vi "ShowDiff.vi"(0 "RawDiff":string, 1 "Alt.Name Old":string, 5 "Alt.Name New":string) -> (6 "UserDone":bool)   [LabVIEW 2013]
uses:
  <vilib>/Utility/miscctls.llb/LVRowAndColumnTypeDef.ctl
  <vilib>/Utility/miscctls.llb/LVRowAndColumnUnsignedTypeDef.ctl
panel:
  in  "Next Button":bool
  in  "Previous Button":bool
  in  "Done":bool
  out "Legend":string[][](table)
  out "FormattedDiff":string[][](table)
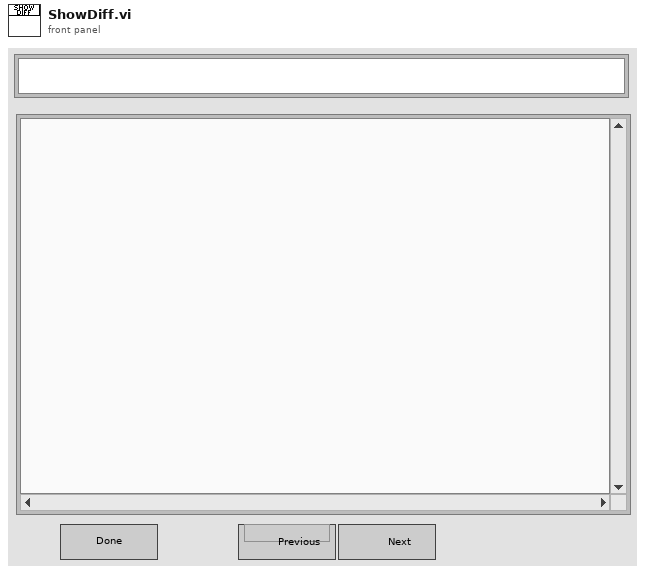
[diagram p1: front panel]
types:
  T1 = typedef "LVRowAndColumnTypeDef.ctl" = cluster{"Row":i32, "Column":i32}
  T2 = cluster{"left":i16, "top":i16, "right":i16, "bottom":i16}
  T3 = typedef "LVRowAndColumnUnsignedTypeDef.ctl" = cluster{"Row":u32, "Column":u32}
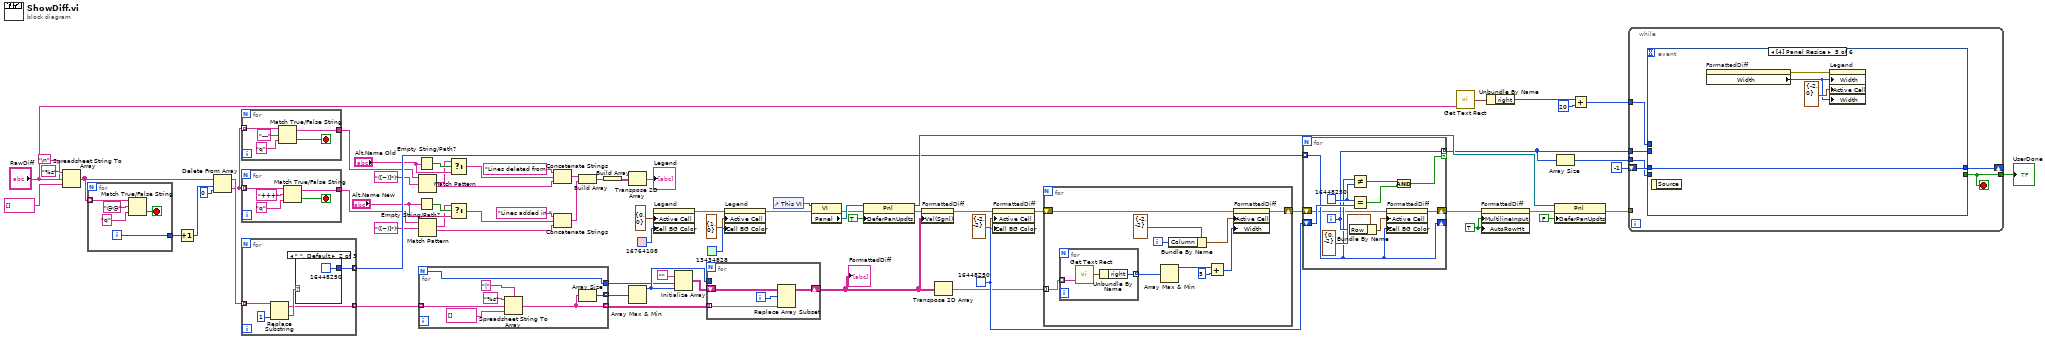
[diagram p0: block diagram]
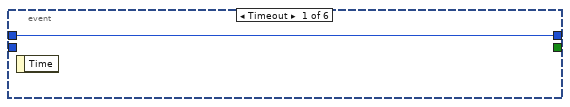
[diagram p2: hidden frame]
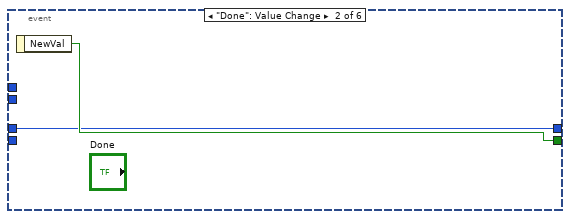
[diagram p3: hidden frame]
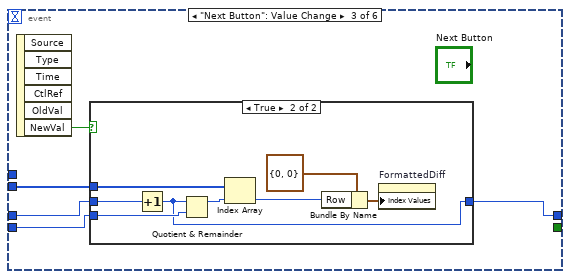
[diagram p4: hidden frame]
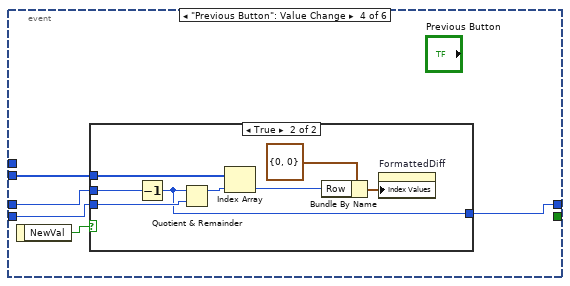
[diagram p6: hidden frame]
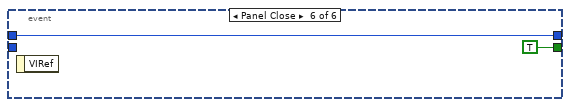
[diagram p8: hidden frame]
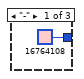
[diagram p9: hidden frame]
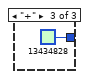
[diagram p10: hidden frame]
diagram:
  w59 = TRUE ("Multiple Line Input")
  w21 = u32 16448250
  n1 = Spreadsheet String To Array(delimiter (Tab)="\n", format string="%s", spreadsheet string="RawDiff", array type (2D Dbl)=string[] []) -> (array=w27:string[])
  n2 = for {
    tunnel: [w76] -> w26
    tunnel: w27 -> [w73] mode=indexing
    i -> [w76]
    stop <- w75 stop-if-true
    n3 = Match True/False String(2:"q" ("false string"), 3:"@@" ("true string"), 4:w73) -> (0:w75:bool)  [unwired: 1 out]
  }
  n4 = Increment(x=w26) -> (x+1=w25:i32)
  n5 = Delete From Array(array=w27, length=w25, index=0) -> (deleted portion=w23:string[], array with subset deleted=w62:string[])
  n6 = for {
    tunnel: w23 -> [w79] mode=indexing
    tunnel: [w77] -> w22
    stop <- w81 stop-if-true
    n7 = Match True/False String(2:"q" ("false string"), 3:"---" ("true string"), 4:w79) -> (0:w81:bool, 1:w77:string)
  }
  n8 = for {
    tunnel: w23 -> [w84] mode=indexing
    tunnel: [w82] -> w24
    stop <- w86 stop-if-true
    n9 = Match True/False String(2:"q" ("false string"), 3:"+++" ("true string"), 4:w84) -> (0:w86:bool, 1:w82:string)
  }
  n10 = for {
    tunnel: w62 -> [w91] mode=indexing
    tunnel: [w89] -> w58 mode=indexing
    tunnel: [w87] -> w13 mode=indexing
    n11 = Replace Substring(2:1 ("length (len. of substring)"), 5:w91) -> (0:w88:string, 1:w87:string)  [unwired: 2 in]
    n12 = case shown="\" \", Default" w88 {
      tunnel: [u32 16764108 u32 16448250 u32 13434828] -> w89
      frame "-" {
      }
      frame " ", Default {
      }
      frame "+" {
      }
    }
  }
  n13 = Empty String/Path?(string/path="Alt.Name Old") -> (empty?=w45:bool)
  n14 = Empty String/Path?(string/path="Alt.Name New") -> (empty?=w36:bool)
  n15 = Match Pattern(string=w22, regular expression="([~)]*)") -> (match substring=w43:string, after substring=w41:string)  [unwired: 1 in, 2 out]
  n16 = Match Pattern(string=w24, regular expression="([~)]*)") -> (match substring=w35:string, after substring=w31:string)  [unwired: 1 in, 2 out]
  n17 = for {
    N -> [w95]
    tunnel: w13 -> [w98] mode=indexing
    tunnel: [w99] -> w12 mode=indexing
    tunnel: [w96] -> w11 mode=indexing
    tunnel: [w95] -> w7
    n18 = Spreadsheet String To Array(delimiter (Tab)="|", format string="%s", spreadsheet string=w98, array type (2D Dbl)=string[] []) -> (array=w96:string[])
    n19 = Array Size(array=w96) -> (size(s)=w99:i32)
  }
  n20 = Select(t=w43, s=w45, f="Alt.Name Old") -> (s? t:f=w42:string)
  n21 = Select(t=w35, s=w36, f="Alt.Name New") -> (s? t:f=w32:string)
  n22 = Concatenate Strings("Lines deleted from " ("string"), w42, w41) -> (w39:string)
  n23 = Concatenate Strings("Lines added in " ("string"), w32, w31) -> (w34:string)
  n24 = Build Array(w39, w34) -> (w28:string[])
  n25 = Build Array(w28) -> (w29:string[][])
  n26 = Transpose 2D Array(2D array=w29) -> (transposed array=→"Legend":string[][])
  n27 = Array Max & Min(array=w12) -> (max value=w8:i32)  [unwired: 3 out]
  n28 = property on="Legend" class="Tbl (strict)"("Active Cell"=T1 {"Row"=0, "Column"=0} ("Active Cell:Active Cell"), "Cell BG Color"=u32 16764108) -> (error out=w47:errorcluster)  [unwired: 2 in, 1 out]
  n29 = Initialize Array("", w7, w8) -> (w9:string[][])
  n30 = for {
    tunnel: w8 -> [_]
    tunnel: w11 -> [w104] mode=indexing
    shift-right: [w102] -> w6
    shift-left: w9 -> [w105]
    i -> [w103]
    n31 = Replace Array Subset(array=w105, new element=w104, index (row)=w103) -> (w102:string[][])  [unwired: 1 in]
  }
  "FormattedDiff" <- w6
  n32 = property on="Legend" class="Tbl (strict)"(error in=w47, "Active Cell"=T1 {"Row"=1, "Column"=0} ("Active Cell:Active Cell"), "Cell BG Color"=u32 13434828) -> (error out=w17:errorcluster)  [unwired: 1 in, 1 out]
  n33 = control-ref of="This VI"() -> (w71:refnum<vi>)
  n34 = property class="VI"(reference=w71, error in=w17) -> (error out=w69:errorcluster, "Panel"=w70:refnum<vi>)  [unwired: 1 out]
  n35 = property on="Property Node" class="Pnl"(reference=w70, error in=w69, "DeferPanUpdts"=TRUE ("Defer Panel Updates")) -> (reference out=w67:refnum<vi>, error out=w14:errorcluster)
  n36 = property on="FormattedDiff" class="Tbl (strict)"(error in=w14, "Val(Sgnl)"=w6) -> (error out=w15:errorcluster)  [unwired: 1 in, 1 out]
  n37 = Transpose 2D Array(2D array=w6) -> (transposed array=w5:string[][])
  n38 = property on="FormattedDiff" class="Tbl (strict)"(error in=w15, "Active Cell"=T1 {"Row"=-2, "Column"=-2} ("Active Cell:Active Cell"), "Cell BG Color"=w21) -> (error out=w3:errorcluster)  [unwired: 1 in, 1 out]
  n39 = for {
    tunnel: w5 -> [w115] mode=indexing
    shift-right: [w106] -> w1
    shift-left: w3 -> [w107]
    i -> [w111]
    n40 = for {
      tunnel: w115 -> [w117] mode=indexing
      tunnel: [w116] -> w114 mode=indexing
      n41 = call <vilib>:"Get Text Rect.vi"("text"=w117) -> ("rect"=w118:T2)  [unwired: 8 in]
      n42 = Unbundle By Name(w118) -> ("right"=w116:i16)
    }
    n43 = Array Max & Min(array=w114) -> (max value=w110:i16)  [unwired: 3 out]
    n44 = Bundle By Name(cluster=T1 {"Row"=-2, "Column"=-2} ("Active Cell:Active Cell"), "Column"=w111) -> (w112:T1)
    n45 = Add(x=w110, y=i16 5) -> (x+y=w109:i16)
    n46 = property on="FormattedDiff" class="Tbl (strict)"(error in=w107, "Active Cell"=w112, "Width"=w109) -> (error out=w106:errorcluster)  [unwired: 1 in, 1 out]
  }
  n47 = for {
    shift-right: [w120] -> w2
    shift-left: w1 -> [w119]
    tunnel: w58 -> [w121] mode=indexing
    shift-right: [w121] -> _
    shift-left: w21 -> [w126]
    tunnel: [w123] -> w19 mode=indexing if=w122
    i -> [w123]
    w127 = u32 16448250
    n48 = Bundle By Name(cluster=T1 {"Row"=0, "Column"=-2} ("Active Cell:Active Cell"), "Row"=w123) -> (w128:T1)
    n49 = Not Equal?(x=w121, y=w127) -> (x != y?=w125:bool)
    n50 = Equal?(x=w127, y=w126) -> (x = y?=w124:bool)
    n51 = property on="FormattedDiff" class="Tbl (strict)"(error in=w119, "Active Cell"=w128, "Cell BG Color"=w121) -> (error out=w120:errorcluster)  [unwired: 1 in, 1 out]
    n52 = And(x=w125, y=w124) -> (x .and. y?=w122:bool)
  }
  n53 = call <vilib>:"Get Text Rect.vi"("text"="RawDiff") -> ("rect"=w54:T2)  [unwired: 8 in]
  n54 = property on="FormattedDiff" class="Tbl (strict)"(error in=w2, "MultilineInput"=w59, "AutoRowHt"=w59) -> (error out=w60:errorcluster)  [unwired: 1 in, 1 out]
  n55 = Unbundle By Name(w54) -> ("right"=w16:i16)
  n56 = property on="Property Node" class="Pnl"(reference=w67, error in=w60, "DeferPanUpdts"=FALSE ("Defer Panel Updates")) -> (error out=w57:errorcluster)  [unwired: 1 out]
  n57 = Array Size(array=w19) -> (size(s)=w18:i32)
  n58 = Add(x=w16, y=i16 20) -> (x+y=w52:i16)
  n59 = while {
    tunnel: w57 -> [_]
    tunnel: [w135] -> w56
    tunnel: w52 -> [w134]
    tunnel: w19 -> [w133]
    tunnel: w18 -> [w131]
    shift-right: [w130] -> _
    shift-left: -1 -> [w132]
    stop <- w135 stop-if-true
    n60 = event shown="[4] Panel Resize" {
      selector: _ -> [_ _ _ _ _ _]
      dyn-events: _ -> [_ _ _ _ _ _]
      timeout: _ -> [_ _ _ _ _ _]
      tunnel: [_ w138 _ _ _ TRUE ("NewVal")] -> w135
      tunnel: w134 -> [_ _ _ _ _ _]
      tunnel: w133 -> [_ _ w143 w157 _ _]
      tunnel: w132 -> [w136 w137 w141 w155 w168 w171]
      tunnel: w131 -> [_ _ w140 w154 _ _]
      tunnel: [w136 w137 w139 w153 w168 w171] -> w130
      event Timeout {
        n61 = event-data() -> ()  [unwired: 1 in, 1 out]
      }
      event "Done": Value Change {
        n62 = event-data() -> ("NewVal"=w138:bool)  [unwired: 1 in]
      }
      event "Next Button": Value Change {
        n63 = event-data() -> ("NewVal"=w142:bool)  [unwired: 1 in, 5 out]
        n64 = case shown="True" w142 {
          tunnel: w143 -> [_ w149]
          tunnel: w141 -> [w144 w148]
          tunnel: w140 -> [_ w147]
          tunnel: [w144 w145] -> w139
          frame False {
          }
          frame True {
            n65 = Increment(x=w148) -> (x+1=w145:i32)
            n66 = Quotient & Remainder(x=w145, y=w147) -> (x-y*floor(x/y)=w146:i32)  [unwired: 1 out]
            n67 = Index Array(array=w149, index=w146) -> (element=w150:i32)
            n68 = Bundle By Name(cluster=T3 {"Row"=0, "Column"=0} ("Index Values"), "Row"=w150) -> (w151:T3)
            n69 = property on="FormattedDiff" class="Tbl (strict)"("Index Values"=w151) -> ()  [unwired: 2 in, 2 out]
          }
        }
      }
      event "Previous Button": Value Change {
        n70 = event-data() -> ("NewVal"=w156:bool)  [unwired: 1 in]
        n71 = case shown="True" w156 {
          tunnel: w157 -> [_ w164]
          tunnel: w155 -> [w158 w160]
          tunnel: w154 -> [_ w162]
          tunnel: [w158 w159] -> w153
          frame False {
          }
          frame True {
            n72 = Decrement(x=w160) -> (x-1=w159:i32)
            n73 = Quotient & Remainder(x=w159, y=w162) -> (x-y*floor(x/y)=w161:i32)  [unwired: 1 out]
            n74 = Index Array(array=w164, index=w161) -> (element=w163:i32)
            n75 = Bundle By Name(cluster=T3 {"Row"=0, "Column"=0} ("Index Values"), "Row"=w163) -> (w165:T3)
            n76 = property on="FormattedDiff" class="Tbl (strict)"("Index Values"=w165) -> ()  [unwired: 2 in, 2 out]
          }
        }
      }
      event Panel Resize {
        n77 = event-data() -> ()  [unwired: 1 in, 1 out]
        n78 = property on="FormattedDiff" class="Tbl (strict)"() -> (error out=w167:errorcluster, "Width"=w169:u32)  [unwired: 2 in, 1 out]
        n79 = property on="Legend" class="Tbl (strict)"(error in=w167, "Width"=w169, "Active Cell"=T1 {"Row"=-2, "Column"=0} ("Active Cell:Active Cell"), "Width"=w169) -> ()  [unwired: 1 in, 2 out]
      }
      event Panel Close {
        n80 = event-data() -> ()  [unwired: 1 in, 1 out]
      }
    }
  }
  "UserDone" <- w56
